vi "main.vi"() -> ()   [LabVIEW 2018]
uses:
  Coef-Temp-.ctl
  Digit.ctl
  Multiplier.ctl
  Tolerance.ctl
  States.ctl
  Data.ctl
  Data Series.ctl
  CSV Series Reader Tester/CSV Series Read.lvlib
panel:
  out "<":dbl
  out "<":dbl
  out "VALUE":dbl
  out "Coef. T.":u32(colorbox)
  out "Tol":u32(colorbox)
  out "Mult":u32(colorbox)
  out "DIG3":u32(colorbox)
  out "DIG2":u32(colorbox)
  out "DIG1":u32(colorbox)
  in  "Tolerance":T1
  in  "Multiplier":T2
  in  "3° Digit":T3
  in  "2° Digit":T3
  in  "1° Digit":T3
  in  "Coef. Temp.":T4
  in  "N° bandas":u8=4 min=4 max=6 step=1
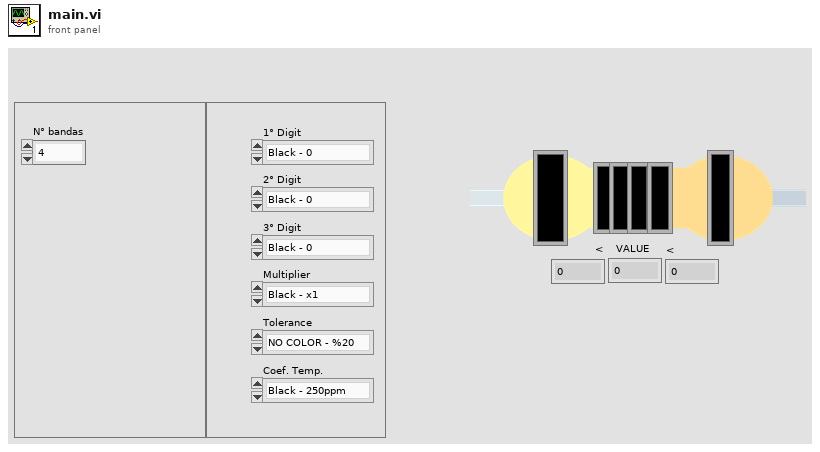
[diagram p1: front panel]
types:
  T1 = typedef "Tolerance.ctl" = enum16{"NO COLOR - %20", "Brown - %1", "Red - %2", "Orange - %3", "Yellow - %4", "Green - %0,5", "Blue - %0,25", "Violet - %0,10", "Grey - %0,05", "Silver x - %10", "Gold x - %5"}
  T2 = typedef "Multiplier.ctl" = enum16{"Black - x1", "Brown - x10", "Red - x100", "Orange - x1.000", "Yellow - x10.000", "Green - x100.000", "Blue - x1.000.000", "Violet -  x 10.000.000", "Grey - x100.000.000", "White - x1.000.000.000", "Silver x - 0,01", "Gold x - 0,1"}
  T3 = typedef "Digit.ctl" = enum16{"Black - 0", "Brown - 1", "Red - 2", "Orange - 3", "Yellow - 4", "Green - 5", "Blue - 6", "Violet - 7", "Grey - 8", "White - 9"}
  T4 = typedef "Coef-Temp-.ctl" = enum16{"Black - 250ppm", "Brown - 100ppm", "Red - 50ppm", "Orange - 15ppm", "Yellow - 25ppm", "Green - 20ppm", "Blue - 10ppm", "Violet - 5ppm"}
  T5 = typedef "Data.ctl" = cluster{"Data Series":T6, "1° Digit":T3, "2° Digit":T3, "3° Digit":T3, "Multiplier":T2, "Tolerance":T1, "Coef. Temp.":T4, "DIG1":u32, "DIG2":u32, "DIG3":u32, "Mult":u32, "Tol":u32, "Coef. T.":u32}
  T6 = typedef "CSV Series Read.lvlib/Data Series.ctl" = cluster{"E3 series":u16[], "E6 series":u16[], "E12 series":u16[], "E24 series":u16[], "E48 series":u16[], "E96 series":u16[], "E192 series":u16[]}
  T7 = typedef "States.ctl" = enum16{"Initialize", "CSV Series Reader ", "Read Parameters", "Set Colors", "Calculate Resistor", "Error", "Shutdown"}
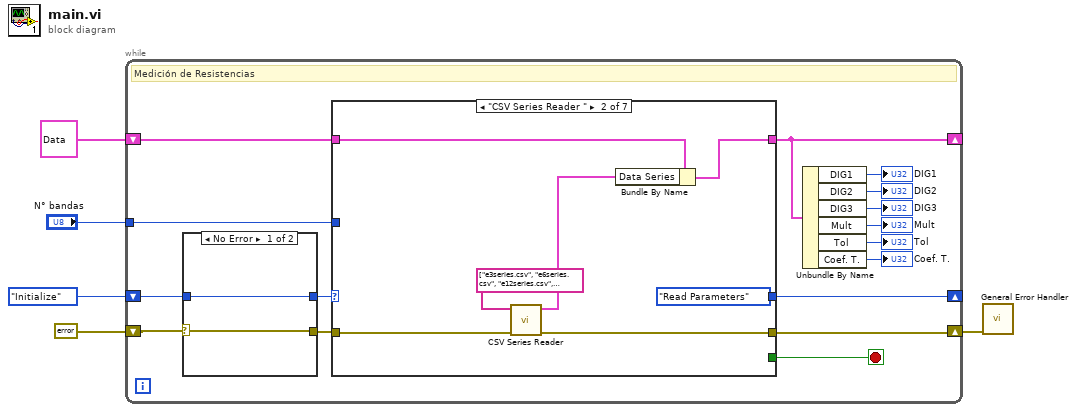
[diagram p0: block diagram]
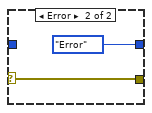
[diagram p2: hidden frame]
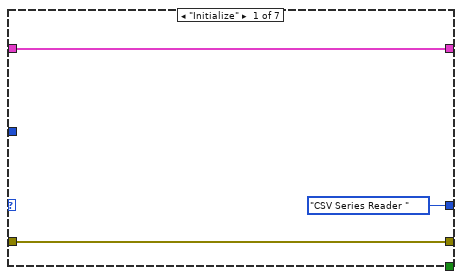
[diagram p3: hidden frame]
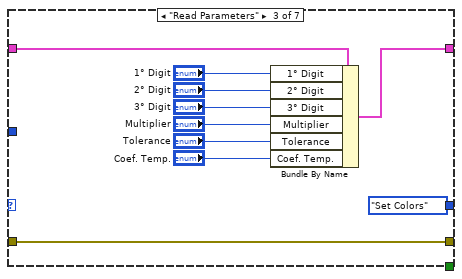
[diagram p4: hidden frame]
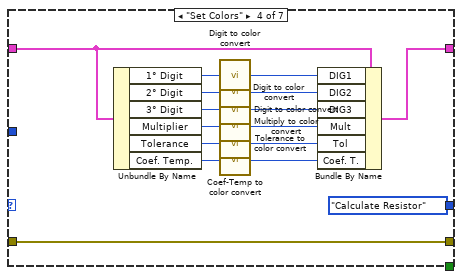
[diagram p5: hidden frame]
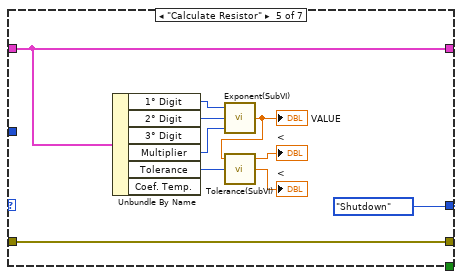
[diagram p6: hidden frame]
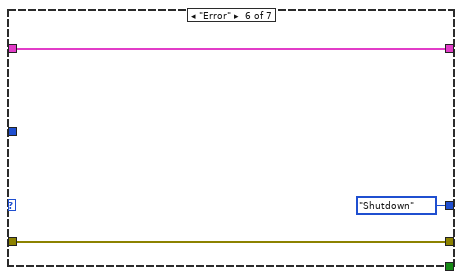
[diagram p7: hidden frame]
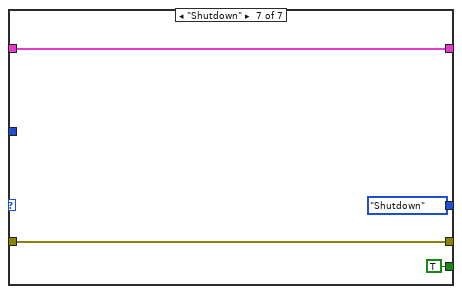
[diagram p8: hidden frame]
diagram:
  n1 = while {
    shift-right: [w15] -> _
    shift-left: States."Initialize" ("States") -> [w19]
    shift-right: [w18] -> w1
    shift-left: errorcluster {"status"=FALSE, "code"=0, "source"=""} ("error in") -> [w17]
    tunnel: "N° bandas" -> [w16]
    shift-right: [w12] -> _
    shift-left: T5 {"Data Series"={"E3 series"=[], "E6 series"=[], "E12 series"=[], "E24 series"=[], "E48 series"=[], "E96 series"=[], "E192 series"=[]}, "1° Digit"=enum."Black - 0", "2° Digit"=enum."Black - 0", "3° Digit"=enum."Black - 0", "Multiplier"=enum."Black - x1", "Tolerance"=enum."NO COLOR - %20", "Coef. Temp."=enum."Black - 250ppm", "DIG1"=0, "DIG2"=0, "DIG3"=0, "Mult"=0, "Tol"=0, "Coef. T."=0} -> [w14]
    stop <- w13 stop-if-true
    # "Medición de Resistencias"
    n2 = case shown="No Error" w17 {
      selector: w17 -> [w22 w25]
      tunnel: w19 -> [w23 _]
      tunnel: [w23 States."Error" ("States")] -> w21
      tunnel: [w22 w25] -> w20
      frame No Error {
      }
      frame Error {
      }
    }
    n3 = case shown="\"CSV Series Reader \"" w21 {
      tunnel: w20 -> [w28 w32 w45 w61 w71 w74 w78]
      tunnel: [w28 w31 w45 w61 w71 w74 w78] -> w18
      tunnel: w16 -> [_ _ _ _ _ _ _]
      tunnel: [States."CSV Series Reader " ("States") States."Read Parameters" ("States") States."Set Colors" ("States") States."Calculate Resistor" ("States") States."Shutdown" ("States") States."Shutdown" ("States") States."Shutdown" ("States")] -> w15
      tunnel: w14 -> [w26 w34 w42 w54 w69 w73 w76]
      tunnel: [w26 w33 w41 w53 w69 w73 w76] -> w12
      tunnel: [_ _ _ _ _ _ TRUE] -> w13
      frame "Initialize" {
      }
      frame "CSV Series Reader " {
        n4 = call "CSV Series Reader.vi"("error in"=w32, "Filenames"=string[] ["e3series.csv", "e6series.csv", "e12series.csv", "e24series.csv", "e48series.csv", "e96series.csv", "e192series.csv"]) -> ("error out"=w31:errorcluster, "Data Series"=w30:T6)  [unwired: 8 in]
        n5 = Bundle By Name(cluster=w34, "Data Series"=w30) -> (w33:T5)
      }
      frame "Read Parameters" {
        n6 = Bundle By Name(cluster=w42, "1° Digit"="1° Digit", "2° Digit"="2° Digit", "3° Digit"="3° Digit", "Multiplier"="Multiplier", "Tolerance"="Tolerance", "Coef. Temp."="Coef. Temp.") -> (w41:T5)
      }
      frame "Set Colors" {
        n7 = Unbundle By Name(w54) -> ("1° Digit"=w46:T3, "2° Digit"=w59:T3, "3° Digit"=w58:T3, "Multiplier"=w57:T2, "Tolerance"=w56:T1, "Coef. Temp."=w55:T4)
        n8 = call "Digit to color convert.vi"("Digit"=w46) -> ("Color Box"=w52:u32)  [unwired: 4 in]
        n9 = call "Digit to color convert.vi"("Digit"=w59) -> ("Color Box"=w51:u32)  [unwired: 4 in]
        n10 = call "Digit to color convert.vi"("Digit"=w58) -> ("Color Box"=w50:u32)  [unwired: 4 in]
        n11 = call "Multiply to color convert.vi"("Multiply"=w57) -> ("Color Box"=w49:u32)  [unwired: 4 in]
        n12 = call "Tolerance to color convert.vi"("Tolerance"=w56) -> ("Color Box"=w48:u32)  [unwired: 4 in]
        n13 = call "Coef-Temp to color convert.vi"("Coef. Temp."=w55) -> ("Color Box"=w47:u32)  [unwired: 4 in]
        n14 = Bundle By Name(cluster=w54, "DIG1"=w52, "DIG2"=w51, "DIG3"=w50, "Mult"=w49, "Tol"=w48, "Coef. T."=w47) -> (w53:T5)
      }
      frame "Calculate Resistor" {
        n15 = Unbundle By Name(w69) -> ("1° Digit"=w68:T3, "2° Digit"=w67:T3, "Multiplier"=w66:T2, "Tolerance"=w62:T1)  [unwired: 2 out]
        n16 = call "Exponent(SubVI).vi"("Multiplier"=w66, "2° Digit"=w67, "1° Digit"=w68) -> ("x*y"=w63:dbl)  [unwired: 2 in]
        "VALUE" <- w63
        n17 = call "Tolerance(SubVI).vi"("Tolerance"=w62, "x*y"=w63) -> ("x-y"=→"<":dbl, "x+y"=→"<":dbl)  [unwired: 2 in]
      }
      frame "Error" {
      }
      frame "Shutdown" {
      }
    }
    n18 = Unbundle By Name(w12) -> ("DIG1"=→"DIG1":u32, "DIG2"=→"DIG2":u32, "DIG3"=→"DIG3":u32, "Mult"=→"Mult":u32, "Tol"=→"Tol":u32, "Coef. T."=→"Coef. T.":u32)
  }
  n19 = call <vilib>:"General Error Handler.vi"("error in (no error)"=w1) -> ()  [unwired: 10 in, 5 out]
